vi "Initialize Small Field.vi"(8 "error in (no error)":errorcluster, 11 "Magna Power in":refnum<class "Magna Power.lvclass">) -> (0 "error out":errorcluster, 2 "Positive?":bool, 3 "Magna Power out":refnum<class "Magna Power.lvclass">)   [LabVIEW 2012, in "Magna Power.lvclass"]
uses:
  Magna Power.lvclass
  Magna Power.lvclass/Magna Power.ctl
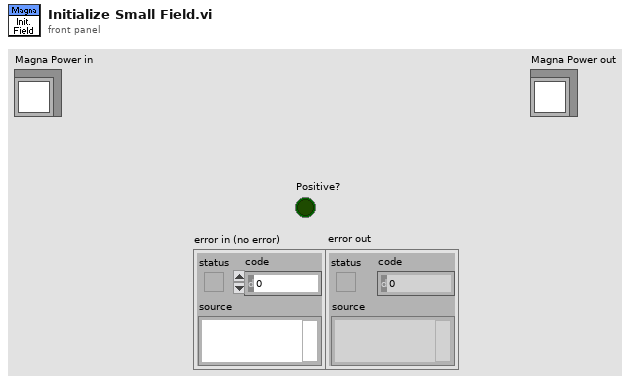
[diagram p1: front panel]
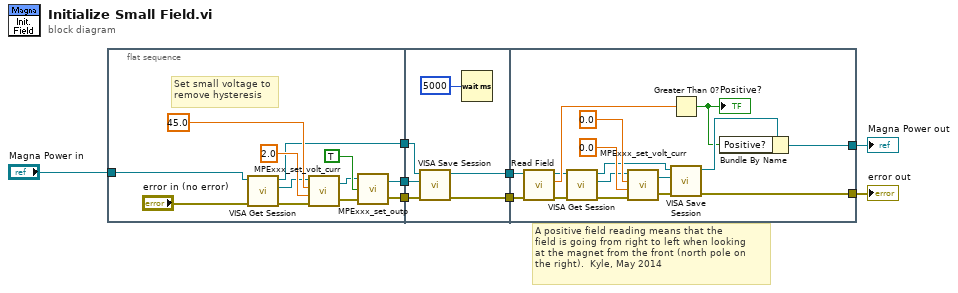
[diagram p0: block diagram]
diagram:
  # "A positive field reading means that the\nfield is going from right to left when looking\nat the magnet from the front (north pole on\nthe right).  Kyle, May 2014"
  n1 = flat-sequence {
    tunnel: [w15] -> w8
    tunnel: [w14] -> w7
    tunnel: "Magna Power in" -> [w12]
    tunnel: [w9] -> w4
    tunnel: w8 -> [w24]
    tunnel: w7 -> [w25]
    tunnel: [w22] -> w6
    tunnel: w4 -> [w23]
    tunnel: [w21] -> w3
    tunnel: [w41] -> w1
    tunnel: [w42] -> w2
    tunnel: w3 -> [w36]
    tunnel: w6 -> [w37]
    frame #0 {
      # "Set small voltage to\nremove hysteresis"
      n2 = call-dynamic "VISA Get Session.vi"("error in (no error)"="error in (no error)", "Instrument.lvclass in"=w12) -> ("error out"=w10:errorcluster, "VISA Resource Name"=w11:refnum<visa-resource-name>, "Instrument.lvclass out"=w9:refnum<class "Magna Power.lvclass">)  [unwired: 6 in, 1 out]
      n3 = call "MPExxx_set_volt_curr.vi"("error in (no error)"=w10, "Set Current"=2.0, "Set Voltage"=45.0, "VISA session"=w11) -> ("error out"=w16:errorcluster, "dup VISA session"=w17:refnum<visa-resource-name>)
      n4 = call "MPExxx_set_outp.vi"("error in (no error)"=w16, "Output Control"=TRUE, "VISA session"=w17) -> ("error out"=w14:errorcluster, "dup VISA session"=w15:refnum<visa-resource-name>)
    }
    frame #1 {
      n5 = call-dynamic "VISA Save Session.vi"("error in (no error)"=w25, "VISA Resource Name"=w24, "Instrument.lvclass in"=w23) -> ("error out"=w22:errorcluster, "Instrument.lvclass out"=w21:refnum<class "Magna Power.lvclass">)  [unwired: 7 in]
      n6 = Wait (ms)(milliseconds to wait=u32 5000) -> ()  [unwired: 1 out]
    }
    frame #2 {
      n7 = call "Read Field.vi"("error in (no error)"=w37, "Magna Power in"=w36) -> ("error out"=w35:errorcluster, "Field (T)"=w38:dbl, "Magna Power out"=w34:refnum<class "Magna Power.lvclass">)  [unwired: 5 in, 2 out]
      n8 = call-dynamic "VISA Get Session.vi"("error in (no error)"=w35, "Instrument.lvclass in"=w34) -> ("error out"=w32:errorcluster, "VISA Resource Name"=w33:refnum<visa-resource-name>, "Instrument.lvclass out"=w31:refnum<class "Magna Power.lvclass">)  [unwired: 6 in, 1 out]
      n9 = call "MPExxx_set_volt_curr.vi"("error in (no error)"=w32, "Set Current"=0.0, "Set Voltage"=0.0, "VISA session"=w33) -> ("error out"=w27:errorcluster, "dup VISA session"=w28:refnum<visa-resource-name>)
      n10 = Greater Than 0?(x=w38) -> (x > 0?=w29:bool)
      "Positive?" <- w29
      n11 = call-dynamic "VISA Save Session.vi"("error in (no error)"=w27, "VISA Resource Name"=w28, "Instrument.lvclass in"=w31) -> ("error out"=w42:errorcluster, "Instrument.lvclass out"=w30:refnum<class "Magna Power.lvclass">)  [unwired: 7 in]
      n12 = Bundle By Name(cluster=w30, "Positive?"=w29) -> (w41:refnum<class "Magna Power.lvclass">)
    }
  }
  "Magna Power out" <- w1
  "error out" <- w2
